vi "S4GUI.vi"(7 "Tab ObsEng":enum32{"Obs", "CCD modes", "Guider", "Eng"}(tab)) -> ()   [LabVIEW 2018] (continued)
                n4865 = Select(t=u8 0, s=w11820, f=u8 6 ("SHUTTER_MODE")) -> (s? t:f=w11821:u8)
              }
            }
          }
          frame Default {
            # "Polar. COM exp mode"
            # "Internal"
            # "Polar. SEM exp mode"
            # "Ext. Start"
            n4866 = Select(t=u8 0, s=w11827, f=u8 6 ("SHUTTER_MODE")) -> (s? t:f=w11824:u8)
          }
        }
        n4867 = call "Write Instrument.lvclass.vi"("error in (no error)"=w11478, "Instrument.lvclass"=w11558, "S4ACS_GUI in"=w11462) -> ("error out"=w11477:errorcluster, "S4ACS_GUI out"=w11466:refnum<class "S4GUI.lvclass">)  [unwired: 7 in]
        n4868 = call-dynamic "Read AcquisitionC.vi"("error in (no error)"=w11477, "S4ACS_GUI in"=w11466) -> ("error out"=w11488:errorcluster, "Acquisition.lvclass"=w11487:refnum<class "Acquisition.lvclass">)  [unwired: 7 in, 1 out]
        n4869 = call-dynamic "Read AcquisitionA.vi"("error in (no error)"=w11477, "S4ACS_GUI in"=w11466) -> ("error out"=w11491:errorcluster, "Acquisition.lvclass"=w11492:refnum<class "Acquisition.lvclass">)  [unwired: 7 in, 1 out]
        n4870 = call "Read AcquisitionB.vi"("error in (no error)"=w11477, "S4ACS_GUI in"=w11466) -> ("error out"=w11489:errorcluster, "Acquisition.lvclass"=w11490:refnum<class "Acquisition.lvclass">)  [unwired: 7 in, 1 out]
        n4871 = call-dynamic "Read AcquisitionD.vi"("error in (no error)"=w11477, "S4ACS_GUI in"=w11466) -> ("error out"=w11485:errorcluster, "Acquisition.lvclass"=w11486:refnum<class "Acquisition.lvclass">)  [unwired: 7 in, 1 out]
        n4872 = call "Read connection.vi"("error in (no error)"=w11488, "Server in"=w11487) -> ("error out"=w11494:errorcluster, "connection"=w11493:bool, "Server out"=w11495:refnum<class "Acquisition.lvclass">)  [unwired: 7 in]
        n4873 = call "Read connection.vi"("error in (no error)"=w11489, "Server in"=w11490) -> ("error out"=w11497:errorcluster, "connection"=w11496:bool, "Server out"=w11498:refnum<class "Acquisition.lvclass">)  [unwired: 7 in]
        n4874 = call "Read connection.vi"("error in (no error)"=w11485, "Server in"=w11486) -> ("error out"=w11474:errorcluster, "connection"=w11475:bool, "Server out"=w11476:refnum<class "Acquisition.lvclass">)  [unwired: 7 in]
        n4875 = call "Read connection.vi"("error in (no error)"=w11491, "Server in"=w11492) -> ("error out"=w11500:errorcluster, "connection"=w11499:bool, "Server out"=w11501:refnum<class "Acquisition.lvclass">)  [unwired: 7 in]
        n4876 = case shown="True" w11493 {
          tunnel: w11495 -> [w11665 w11670]
          tunnel: w11494 -> [w11664 w11669]
          tunnel: [w11665 w11668] -> w11480
          tunnel: [w11664 w11667] -> w11479
          tunnel: w11473 -> [_ w11666]
          frame False {
          }
          frame True {
            # "nome do arquivo .cfg"
            # "seção no arquivo .cfg"
            n4877 = call-dynamic "Read Channel.vi"("error in (no error)"=w11669, "Acquisition in"=w11670) -> ("error out"=w11674:errorcluster, "Channel.lvclass"=w11673:refnum<class "Channel.lvclass">, "Acquisition out"=w11672:refnum<class "Acquisition.lvclass">)  [unwired: 7 in]
            n4878 = call-dynamic "Read Interface.vi"("error in (no error)"=w11674, "Channel in"=w11673) -> ("error out"=w11681:errorcluster, "Interface.lvclass"=w11682:refnum<class "Interface.lvclass">, "Channel out"=w11671:refnum<class "Channel.lvclass">)  [unwired: 7 in]
            n4879 = call-dynamic "Get CCD_Config.vi"("error in (no error)"=w11681, "Interface in"=w11682) -> ("error out"=w11679:errorcluster, "output cluster"=w11678:T31, "Interface out"=w11683:refnum<class "Interface.lvclass">)  [unwired: 7 in]
            n4880 = Bundle By Name(cluster=w11678, "TRIGGER_MODE"=w11666) -> (w11680:T31)
            n4881 = call-dynamic "Set CCD_Config.vi"("error in (no error)"=w11679, "input cluster"=w11680, "Interface in"=w11683) -> ("error out"=w11677:errorcluster, "Interface out"=w11684:refnum<class "Interface.lvclass">)  [unwired: 7 in]
            n4882 = Flatten To String(anything=w11680, error in (no error)=w11677) -> (data string=w11675:string, error out=w11676:errorcluster)  [unwired: 2 in, 1 out]
            n4883 = call "Write flatted cluster.vi"("error in (no error)"=w11676, "flatted cluster"=w11675, "Interface in"=w11684) -> ("error out"=w11686:errorcluster, "Interface out"=w11685:refnum<class "Interface.lvclass">)  [unwired: 7 in]
            n4884 = call-dynamic "Write Interface.vi"("error in (no error)"=w11686, "Interface.lvclass"=w11685, "Channel in"=w11671) -> ("error out"=w11692:errorcluster, "Channel out"=w11693:refnum<class "Channel.lvclass">)  [unwired: 7 in]
            n4885 = call "Write section_name.vi"("error in (no error)"=w11692, "section_name"="CCD_ACS3", "Channel in"=w11693) -> ("error out"=w11690:errorcluster, "Channel out"=w11696:refnum<class "Channel.lvclass">)  [unwired: 7 in]
            n4886 = call-dynamic "save config.vi"("error in (no error)"=w11690, "file config"="lastsaved.cfg", "Channel in"=w11696) -> ("error out"=w11691:errorcluster, "Channel out"=w11697:refnum<class "Channel.lvclass">)  [unwired: 7 in]
            n4887 = call-dynamic "Read State Machine.vi"("error in (no error)"=w11691, "Device in"=w11697) -> ("error out"=w11687:errorcluster, "State Machine.lvclass"=w11699:refnum<class "State Machine.lvclass">, "Device out"=w11698:refnum<class "Channel.lvclass">)  [unwired: 7 in]
            n4888 = call-dynamic "Write State.vi"("error in (no error)"=w11687, "State"=60, "State Machine in"=w11699) -> ("error out"=w11688:errorcluster, "State Machine out"=w11700:refnum<class "State Machine.lvclass">)  [unwired: 7 in]
            n4889 = call-dynamic "Write State Machine.vi"("error in (no error)"=w11688, "State Machine.lvclass"=w11700, "Device in"=w11698) -> ("error out"=w11702:errorcluster, "Device out"=w11701:refnum<class "Channel.lvclass">)  [unwired: 7 in]
            n4890 = call-dynamic "Write Channel.vi"("error in (no error)"=w11702, "Channel.lvclass"=w11701, "Acquisition in"=w11672) -> ("error out"=w11667:errorcluster, "Acquisition out"=w11668:refnum<class "Acquisition.lvclass">)  [unwired: 7 in]
          }
        }
        n4891 = case shown="True" w11475 {
          tunnel: w11476 -> [w11626 w11631]
          tunnel: w11474 -> [w11625 w11630]
          tunnel: w11473 -> [_ w11629]
          tunnel: [w11626 w11628] -> w11472
          tunnel: [w11625 w11627] -> w11471
          frame False {
          }
          frame True {
            # "nome do arquivo .cfg"
            # "seção no arquivo .cfg"
            n4892 = call-dynamic "Read Channel.vi"("error in (no error)"=w11630, "Acquisition in"=w11631) -> ("error out"=w11660:errorcluster, "Channel.lvclass"=w11661:refnum<class "Channel.lvclass">, "Acquisition out"=w11662:refnum<class "Acquisition.lvclass">)  [unwired: 7 in]
            n4893 = call-dynamic "Read Interface.vi"("error in (no error)"=w11660, "Channel in"=w11661) -> ("error out"=w11653:errorcluster, "Interface.lvclass"=w11652:refnum<class "Interface.lvclass">, "Channel out"=w11663:refnum<class "Channel.lvclass">)  [unwired: 7 in]
            n4894 = call-dynamic "Get CCD_Config.vi"("error in (no error)"=w11653, "Interface in"=w11652) -> ("error out"=w11655:errorcluster, "output cluster"=w11656:T31, "Interface out"=w11651:refnum<class "Interface.lvclass">)  [unwired: 7 in]
            n4895 = Bundle By Name(cluster=w11656, "TRIGGER_MODE"=w11629) -> (w11654:T31)
            n4896 = call-dynamic "Set CCD_Config.vi"("error in (no error)"=w11655, "input cluster"=w11654, "Interface in"=w11651) -> ("error out"=w11657:errorcluster, "Interface out"=w11650:refnum<class "Interface.lvclass">)  [unwired: 7 in]
            n4897 = Flatten To String(anything=w11654, error in (no error)=w11657) -> (data string=w11659:string, error out=w11658:errorcluster)  [unwired: 2 in, 1 out]
            n4898 = call "Write flatted cluster.vi"("error in (no error)"=w11658, "flatted cluster"=w11659, "Interface in"=w11650) -> ("error out"=w11648:errorcluster, "Interface out"=w11649:refnum<class "Interface.lvclass">)  [unwired: 7 in]
            n4899 = call-dynamic "Write Interface.vi"("error in (no error)"=w11648, "Interface.lvclass"=w11649, "Channel in"=w11663) -> ("error out"=w11642:errorcluster, "Channel out"=w11641:refnum<class "Channel.lvclass">)  [unwired: 7 in]
            n4900 = call "Write section_name.vi"("error in (no error)"=w11642, "section_name"="CCD_ACS4", "Channel in"=w11641) -> ("error out"=w11644:errorcluster, "Channel out"=w11638:refnum<class "Channel.lvclass">)  [unwired: 7 in]
            n4901 = call-dynamic "save config.vi"("error in (no error)"=w11644, "file config"="lastsaved.cfg", "Channel in"=w11638) -> ("error out"=w11643:errorcluster, "Channel out"=w11637:refnum<class "Channel.lvclass">)  [unwired: 7 in]
            n4902 = call-dynamic "Read State Machine.vi"("error in (no error)"=w11643, "Device in"=w11637) -> ("error out"=w11647:errorcluster, "State Machine.lvclass"=w11635:refnum<class "State Machine.lvclass">, "Device out"=w11636:refnum<class "Channel.lvclass">)  [unwired: 7 in]
            n4903 = call-dynamic "Write State.vi"("error in (no error)"=w11647, "State"=60, "State Machine in"=w11635) -> ("error out"=w11646:errorcluster, "State Machine out"=w11634:refnum<class "State Machine.lvclass">)  [unwired: 7 in]
            n4904 = call-dynamic "Write State Machine.vi"("error in (no error)"=w11646, "State Machine.lvclass"=w11634, "Device in"=w11636) -> ("error out"=w11632:errorcluster, "Device out"=w11633:refnum<class "Channel.lvclass">)  [unwired: 7 in]
            n4905 = call-dynamic "Write Channel.vi"("error in (no error)"=w11632, "Channel.lvclass"=w11633, "Acquisition in"=w11662) -> ("error out"=w11627:errorcluster, "Acquisition out"=w11628:refnum<class "Acquisition.lvclass">)  [unwired: 7 in]
          }
        }
        n4906 = case shown="True" w11496 {
          tunnel: w11498 -> [w11704 w11709]
          tunnel: w11497 -> [w11703 w11708]
          tunnel: [w11704 w11707] -> w11482
          tunnel: [w11703 w11706] -> w11481
          tunnel: w11473 -> [_ w11705]
          frame False {
          }
          frame True {
            # "nome do arquivo .cfg"
            # "seção no arquivo .cfg"
            n4907 = call-dynamic "Read Channel.vi"("error in (no error)"=w11708, "Acquisition in"=w11709) -> ("error out"=w11713:errorcluster, "Channel.lvclass"=w11712:refnum<class "Channel.lvclass">, "Acquisition out"=w11711:refnum<class "Acquisition.lvclass">)  [unwired: 7 in]
            n4908 = call-dynamic "Read Interface.vi"("error in (no error)"=w11713, "Channel in"=w11712) -> ("error out"=w11720:errorcluster, "Interface.lvclass"=w11721:refnum<class "Interface.lvclass">, "Channel out"=w11710:refnum<class "Channel.lvclass">)  [unwired: 7 in]
            n4909 = call-dynamic "Get CCD_Config.vi"("error in (no error)"=w11720, "Interface in"=w11721) -> ("error out"=w11718:errorcluster, "output cluster"=w11717:T31, "Interface out"=w11722:refnum<class "Interface.lvclass">)  [unwired: 7 in]
            n4910 = Bundle By Name(cluster=w11717, "TRIGGER_MODE"=w11705) -> (w11719:T31)
            n4911 = call-dynamic "Set CCD_Config.vi"("error in (no error)"=w11718, "input cluster"=w11719, "Interface in"=w11722) -> ("error out"=w11716:errorcluster, "Interface out"=w11723:refnum<class "Interface.lvclass">)  [unwired: 7 in]
            n4912 = Flatten To String(anything=w11719, error in (no error)=w11716) -> (data string=w11714:string, error out=w11715:errorcluster)  [unwired: 2 in, 1 out]
            n4913 = call "Write flatted cluster.vi"("error in (no error)"=w11715, "flatted cluster"=w11714, "Interface in"=w11723) -> ("error out"=w11725:errorcluster, "Interface out"=w11724:refnum<class "Interface.lvclass">)  [unwired: 7 in]
            n4914 = call-dynamic "Write Interface.vi"("error in (no error)"=w11725, "Interface.lvclass"=w11724, "Channel in"=w11710) -> ("error out"=w11731:errorcluster, "Channel out"=w11732:refnum<class "Channel.lvclass">)  [unwired: 7 in]
            n4915 = call "Write section_name.vi"("error in (no error)"=w11731, "section_name"="CCD_ACS2", "Channel in"=w11732) -> ("error out"=w11729:errorcluster, "Channel out"=w11735:refnum<class "Channel.lvclass">)  [unwired: 7 in]
            n4916 = call-dynamic "save config.vi"("error in (no error)"=w11729, "file config"="lastsaved.cfg", "Channel in"=w11735) -> ("error out"=w11730:errorcluster, "Channel out"=w11736:refnum<class "Channel.lvclass">)  [unwired: 7 in]
            n4917 = call-dynamic "Read State Machine.vi"("error in (no error)"=w11730, "Device in"=w11736) -> ("error out"=w11726:errorcluster, "State Machine.lvclass"=w11738:refnum<class "State Machine.lvclass">, "Device out"=w11737:refnum<class "Channel.lvclass">)  [unwired: 7 in]
            n4918 = call-dynamic "Write State.vi"("error in (no error)"=w11726, "State"=60, "State Machine in"=w11738) -> ("error out"=w11727:errorcluster, "State Machine out"=w11739:refnum<class "State Machine.lvclass">)  [unwired: 7 in]
            n4919 = call-dynamic "Write State Machine.vi"("error in (no error)"=w11727, "State Machine.lvclass"=w11739, "Device in"=w11737) -> ("error out"=w11741:errorcluster, "Device out"=w11740:refnum<class "Channel.lvclass">)  [unwired: 7 in]
            n4920 = call-dynamic "Write Channel.vi"("error in (no error)"=w11741, "Channel.lvclass"=w11740, "Acquisition in"=w11711) -> ("error out"=w11706:errorcluster, "Acquisition out"=w11707:refnum<class "Acquisition.lvclass">)  [unwired: 7 in]
          }
        }
        n4921 = case shown="True" w11499 {
          tunnel: [w11742 w11776] -> w11483
          tunnel: [w11743 w11775] -> w11484
          tunnel: w11501 -> [w11743 w11746]
          tunnel: w11500 -> [w11742 w11745]
          tunnel: w11473 -> [_ w11744]
          frame False {
          }
          frame True {
            # "nome do arquivo .cfg"
            # "seção no arquivo .cfg"
            n4922 = call-dynamic "Read Channel.vi"("error in (no error)"=w11745, "Acquisition in"=w11746) -> ("error out"=w11777:errorcluster, "Channel.lvclass"=w11778:refnum<class "Channel.lvclass">, "Acquisition out"=w11779:refnum<class "Acquisition.lvclass">)  [unwired: 7 in]
            n4923 = call-dynamic "Read Interface.vi"("error in (no error)"=w11777, "Channel in"=w11778) -> ("error out"=w11768:errorcluster, "Interface.lvclass"=w11767:refnum<class "Interface.lvclass">, "Channel out"=w11780:refnum<class "Channel.lvclass">)  [unwired: 7 in]
            n4924 = call-dynamic "Get CCD_Config.vi"("error in (no error)"=w11768, "Interface in"=w11767) -> ("error out"=w11770:errorcluster, "output cluster"=w11771:T31, "Interface out"=w11766:refnum<class "Interface.lvclass">)  [unwired: 7 in]
            n4925 = Bundle By Name(cluster=w11771, "TRIGGER_MODE"=w11744) -> (w11769:T31)
            n4926 = call-dynamic "Set CCD_Config.vi"("error in (no error)"=w11770, "input cluster"=w11769, "Interface in"=w11766) -> ("error out"=w11772:errorcluster, "Interface out"=w11765:refnum<class "Interface.lvclass">)  [unwired: 7 in]
            n4927 = Flatten To String(anything=w11769, error in (no error)=w11772) -> (data string=w11774:string, error out=w11773:errorcluster)  [unwired: 2 in, 1 out]
            n4928 = call "Write flatted cluster.vi"("error in (no error)"=w11773, "flatted cluster"=w11774, "Interface in"=w11765) -> ("error out"=w11763:errorcluster, "Interface out"=w11764:refnum<class "Interface.lvclass">)  [unwired: 7 in]
            n4929 = call-dynamic "Write Interface.vi"("error in (no error)"=w11763, "Interface.lvclass"=w11764, "Channel in"=w11780) -> ("error out"=w11758:errorcluster, "Channel out"=w11757:refnum<class "Channel.lvclass">)  [unwired: 7 in]
            n4930 = call "Write section_name.vi"("error in (no error)"=w11758, "section_name"="CCD_ACS1", "Channel in"=w11757) -> ("error out"=w11759:errorcluster, "Channel out"=w11754:refnum<class "Channel.lvclass">)  [unwired: 7 in]
            n4931 = call-dynamic "save config.vi"("error in (no error)"=w11759, "file config"="lastsaved.cfg", "Channel in"=w11754) -> ("error out"=w11747:errorcluster, "Channel out"=w11748:refnum<class "Channel.lvclass">)  [unwired: 7 in]
            n4932 = call-dynamic "Read State Machine.vi"("error in (no error)"=w11747, "Device in"=w11748) -> ("error out"=w11762:errorcluster, "State Machine.lvclass"=w11752:refnum<class "State Machine.lvclass">, "Device out"=w11753:refnum<class "Channel.lvclass">)  [unwired: 7 in]
            n4933 = call-dynamic "Write State.vi"("error in (no error)"=w11762, "State"=60, "State Machine in"=w11752) -> ("error out"=w11761:errorcluster, "State Machine out"=w11751:refnum<class "State Machine.lvclass">)  [unwired: 7 in]
            n4934 = call-dynamic "Write State Machine.vi"("error in (no error)"=w11761, "State Machine.lvclass"=w11751, "Device in"=w11753) -> ("error out"=w11749:errorcluster, "Device out"=w11750:refnum<class "Channel.lvclass">)  [unwired: 7 in]
            n4935 = call-dynamic "Write Channel.vi"("error in (no error)"=w11749, "Channel.lvclass"=w11750, "Acquisition in"=w11779) -> ("error out"=w11776:errorcluster, "Acquisition out"=w11775:refnum<class "Acquisition.lvclass">)  [unwired: 7 in]
          }
        }
        n4936 = call-dynamic "Write AcquisitionA.vi"("error in (no error)"=w11483, "Acquisition.lvclass"=w11484, "S4ACS_GUI in"=w11466) -> ("error out"=w11470:errorcluster, "S4ACS_GUI out"=w11465:refnum<class "S4GUI.lvclass">)  [unwired: 7 in]
        n4937 = call "Write AcquisitionB.vi"("error in (no error)"=w11481, "Acquisition.lvclass"=w11482, "S4ACS_GUI in"=w11465) -> ("error out"=w11469:errorcluster, "S4ACS_GUI out"=w11464:refnum<class "S4GUI.lvclass">)  [unwired: 7 in]
        n4938 = call-dynamic "Write AcquisitionC.vi"("error in (no error)"=w11479, "Acquisition.lvclass"=w11480, "S4ACS_GUI in"=w11464) -> ("error out"=w11468:errorcluster, "S4ACS_GUI out"=w11463:refnum<class "S4GUI.lvclass">)  [unwired: 7 in]
        n4939 = call-dynamic "Write AcquisitionD.vi"("error in (no error)"=w11471, "Acquisition.lvclass"=w11472, "S4ACS_GUI in"=w11463) -> ("error out"=w11467:errorcluster, "S4ACS_GUI out"=w11447:refnum<class "S4GUI.lvclass">)  [unwired: 7 in]
        n4940 = Merge Errors(w11470, w11469, w11468, w11467) -> (w11446:errorcluster)
        n4941 = call "Read Instrument.lvclass.vi"("error in (no error)"=w11446, "S4ACS_GUI in"=w11447) -> ("error out"=w11452:errorcluster, "Instrument.lvclass"=w11451:refnum<class "Instrument.lvclass">, "S4ACS_GUI out"=w11448:refnum<class "S4GUI.lvclass">)  [unwired: 7 in]
        n4942 = call "Read ASEL.vi"("error in (no error)"=w11452, "Instrument in"=w11451) -> ("error out"=w11459:errorcluster, "Opt_Selector.lvclass"=w11458:refnum<class "Opt_Selector.lvclass">, "Instrument out"=w11457:refnum<class "Instrument.lvclass">)  [unwired: 7 in]
        n4943 = call "Read target name.vi"("error in (no error)"=w11459, "Optics in"=w11458) -> ("error out"=w11455:errorcluster, "target name"=w11435:string, "Optics out"=w11456:refnum<class "Opt_Selector.lvclass">)  [unwired: 7 in]
        n4944 = call "Write ASEL.vi"("error in (no error)"=w11455, "Opt_Selector.lvclass"=w11456, "Instrument in"=w11457) -> ("error out"=w11454:errorcluster, "Instrument out"=w11450:refnum<class "Instrument.lvclass">)  [unwired: 7 in]
        n4945 = Concatenate Strings(w11437, " ASEL=" ("string"), w11435) -> (w11432:string)
        n4946 = case shown="\"ON\"" w11435 {
          tunnel: w11454 -> [w11601 w11612]
          tunnel: [w11601 w11608] -> w11453
          tunnel: w11450 -> [w11600 w11613]
          tunnel: [w11600 w11609] -> w11449
          frame Default {
          }
          frame "ON" {
            n4947 = call "Read WPROT.vi"("error in (no error)"=w11612, "Instrument in"=w11613) -> ("error out"=w11604:errorcluster, "Opt_Selector.lvclass"=w11611:refnum<class "Opt_Selector.lvclass">, "Instrument out"=w11610:refnum<class "Instrument.lvclass">)  [unwired: 7 in]
            n4948 = call-dynamic "Read sequencia.vi"("error in (no error)"=w11604, "Opt_Selector in"=w11611) -> ("error out"=w11603:errorcluster, "sequencia"=w11607:u16, "Opt_Selector out"=w11606:refnum<class "Opt_Selector.lvclass">)  [unwired: 7 in]
            n4949 = case shown="0" w11607 {
              tunnel: w11606 -> [w11615 w11624]
              tunnel: [w11615 w11620] -> w11605
              tunnel: w11603 -> [w11614 w11623]
              tunnel: [w11614 w11618] -> w11602
              frame Default {
              }
              frame 0 {
                n4950 = call-dynamic "Write sequencia.vi"("error in (no error)"=w11623, "sequencia"=u16 1, "Opt_Selector in"=w11624) -> ("error out"=w11619:errorcluster, "Opt_Selector out"=w11621:refnum<class "Opt_Selector.lvclass">)  [unwired: 7 in]
                n4951 = local write "P0"(TRUE ("P0")) -> ()
                n4952 = call-dynamic "Write sequencia_ant.vi"("error in (no error)"=w11619, "sequencia_ant"=u16 1, "Opt_Selector in"=w11621) -> ("error out"=w11618:errorcluster, "Opt_Selector out"=w11620:refnum<class "Opt_Selector.lvclass">)  [unwired: 7 in]
              }
            }
            n4953 = call "Write WPROT.vi"("error in (no error)"=w11602, "Opt_Selector.lvclass"=w11605, "Instrument in"=w11610) -> ("error out"=w11608:errorcluster, "Instrument out"=w11609:refnum<class "Instrument.lvclass">)  [unwired: 7 in]
          }
        }
        n4954 = call "Write Instrument.lvclass.vi"("error in (no error)"=w11453, "Instrument.lvclass"=w11449, "S4ACS_GUI in"=w11448) -> ("error out"=w11433:errorcluster, "S4ACS_GUI out"=w11434:refnum<class "S4GUI.lvclass">)  [unwired: 7 in]
        n4955 = call-dynamic "Write User Event.vi"("error in (no error)"=w11433, "User Event"=w11432, "S4GUI in"=w11434) -> ("error out"=w11430:errorcluster, "S4GUI out"=w11431:refnum<class "S4GUI.lvclass">)  [unwired: 7 in]
      }
      event "Init mode": Value Change {
        n4956 = event-data() -> ()  [unwired: 1 in, 4 out]
        n4957 = call-dynamic "Write User Event.vi"("error in (no error)"=w11833, "User Event"="INIT INSTRUMENT CLICKED", "S4GUI in"=w11834) -> ("error out"=w11831:errorcluster, "S4GUI out"=w11832:refnum<class "S4GUI.lvclass">)  [unwired: 7 in]
        n4958 = call-dynamic "Read Obs_state.vi"("error in (no error)"=w11831, "S4ACS_GUI in"=w11832) -> ("error out"=w11835:errorcluster, "Obs_state"=w11837:u32, "S4ACS_GUI out"=w11838:refnum<class "S4GUI.lvclass">)  [unwired: 7 in]
        n4959 = In Range and Coerce(upper limit=u32 226, x=w11837, lower limit=u32 220 ("upper limit")) -> (In Range?=w11836:bool)  [unwired: 1 out]
        n4960 = case shown="False" w11836 {
          tunnel: [w11846 w11854] -> w11842
          tunnel: [w11845 w11852] -> w11841
          tunnel: w11835 -> [w11844 w11853]
          tunnel: w11838 -> [w11843 w11855]
          frame False {
            n4961 = call-dynamic "Write sync.vi"("error in (no error)"=w11844, "sync"=TRUE, "S4ACS_GUI in"=w11843) -> ("error out"=w11848:errorcluster, "S4ACS_GUI out"=w11847:refnum<class "S4GUI.lvclass">)  [unwired: 7 in]
            n4962 = call-dynamic "Write Obs_state.vi"("error in (no error)"=w11848, "Obs_state"=u32 220, "S4ACS_GUI in"=w11847) -> ("error out"=w11845:errorcluster, "S4ACS_GUI out"=w11846:refnum<class "S4GUI.lvclass">)  [unwired: 7 in]
          }
          frame True {
            n4963 = call-dynamic "Write Obs_state.vi"("error in (no error)"=w11853, "Obs_state"=u32 0, "S4ACS_GUI in"=w11855) -> ("error out"=w11852:errorcluster, "S4ACS_GUI out"=w11854:refnum<class "S4GUI.lvclass">)  [unwired: 7 in]
          }
        }
      }
      event "exit": Value Change {
        n4964 = event-data() -> ()  [unwired: 1 in, 4 out]
        n4965 = call-dynamic "Read Obs_state.vi"("error in (no error)"=w11859, "S4ACS_GUI in"=w11860) -> ("error out"=w11857:errorcluster, "Obs_state"=w11861:u32, "S4ACS_GUI out"=w11858:refnum<class "S4GUI.lvclass">)  [unwired: 7 in]
        n4966 = In Range and Coerce(upper limit=u32 239, x=w11861, lower limit=u32 230 ("upper limit")) -> (In Range?=w11856:bool)  [unwired: 1 out]
        n4967 = case shown="False" w11856 {
          tunnel: [w11874 w12006] -> w11865
          tunnel: [w11873 w12005] -> w11864
          tunnel: w11858 -> [w11867 w12006]
          tunnel: w11857 -> [w11866 w12005]
          frame False {
            n4968 = call "Read Instrument.lvclass.vi"("error in (no error)"=w11866, "S4ACS_GUI in"=w11867) -> ("error out"=w11868:errorcluster, "Instrument.lvclass"=w11870:refnum<class "Instrument.lvclass">, "S4ACS_GUI out"=w11872:refnum<class "S4GUI.lvclass">)  [unwired: 7 in]
            n4969 = call-dynamic "Read operational.vi"("error in (no error)"=w11868, "Server in"=w11870) -> ("error out"=w11871:errorcluster, "operational"=w11869:bool)  [unwired: 7 in, 1 out]
            n4970 = case shown="True" w11869 {
              tunnel: [w11884 w11952] -> w11874
              tunnel: [w11883 w11951] -> w11873
              tunnel: w11872 -> [w11881 w11950]
              tunnel: w11871 -> [w11882 w11949]
              frame False {
                # "Park condition:\nidle: T\nAND\nall discon: F"
                # "S4ICS not operational: only ACS parking can \nbe allowed, depending on its status..."
                n4971 = call-dynamic "VerifyAcqStatus.vi"("error in (no error)"=w11882, "S4GUI in"=w11881) -> ("error out"=w11876:errorcluster, "idle"=w11880:bool, "S4GUI out"=w11878:refnum<class "S4GUI.lvclass">)  [unwired: 6 in, 1 out]
                n4972 = case shown="True" w11880 {
                  selector: w11880 -> [w11885 _]
                  tunnel: [w11885 w11888] -> w11879
                  tunnel: w11878 -> [w11887 w11892]
                  tunnel: [w11887 w11891] -> w11877
                  tunnel: w11876 -> [w11886 w11890]
                  tunnel: [w11886 w11889] -> w11875
                  frame False {
                  }
                  frame True {
                    n4973 = call-dynamic "VerifAllChanDiscon.vi"("error in (no error)"=w11890, "S4GUI in"=w11892) -> ("error out"=w11889:errorcluster, "All disconnected"=w11893:bool, "S4GUI out"=w11891:refnum<class "S4GUI.lvclass">)  [unwired: 7 in]
                    n4974 = Not(x=w11893) -> (.not. x?=w11888:bool)
                  }
                }
                n4975 = case shown="False" w11879 {
                  tunnel: w11875 -> [w11902 w11921]
                  tunnel: w11877 -> [w11903 w11920]
                  tunnel: [w11896 w11919] -> w11884
                  tunnel: [w11895 w11918] -> w11883
                  frame False {
                    # "Acquisition in progress OR no channel operational..."
                    n4976 = Two Button Dialog(message="Parking not possible.\nAre you sure to quit?", 2:"Yes" ("T button name (\"OK\")")) -> (T button?=w11899:bool)  [unwired: 1 in]
                    n4977 = case shown="True" w11899 {
                      tunnel: [w11906 w11910] -> w11898
                      tunnel: w11903 -> [w11906 w11911]
                      tunnel: w11902 -> [w11905 w11909]
                      tunnel: [w11905 w11908] -> w11897
                      tunnel: ["EXIT CLICKED WITH NO PARKING POSSIBLE. EXIT CANCELLED. " ("T button name (\"OK\")") "EXIT CLICKED WITH NO PARKING POSSIBLE." ("T button name (\"OK\")")] -> w11894
                      frame False {
                        # "NO (cancel)"
                      }
                      frame True {
                        # "YES"
                        n4978 = call-dynamic "Write exit.vi"("error in (no error)"=w11909, "exit"=TRUE, "S4GUI in"=w11911) -> ("error out"=w11908:errorcluster, "S4GUI out"=w11910:refnum<class "S4GUI.lvclass">)  [unwired: 7 in]
                      }
                    }
                    n4979 = call-dynamic "Write User Event.vi"("error in (no error)"=w11897, "User Event"=w11894, "S4GUI in"=w11898) -> ("error out"=w11895:errorcluster, "S4GUI out"=w11896:refnum<class "S4GUI.lvclass">)  [unwired: 7 in]
                  }
                  frame True {
                    # "No acquisition in progress."
                    n4980 = call <vilib>:"Three Button Dialog.vi"("Right Button Text (\"Cancel\")"="Cancel" ("Right Button Text (\"Cancel\")"), "Center Button Text (\"No\")"="NO" ("F button name (\"Cancel\")"), "Left Button Text (\"Yes\")"="YES" ("T button name (\"OK\")"), "message"="Instrument parking not possible.\nPark acquisition system before exiting?") -> ("Which Button?"=w11916:T34)  [unwired: 7 in]
                    n4981 = case shown="\"Right Button\", Default" w11916 {
                      tunnel: w11921 -> [w11928 w11932 w11941]
                      tunnel: w11920 -> [w11927 w11933 w11940]
                      tunnel: [w11924 w11931 w11937] -> w11919
                      tunnel: [w11922 w11930 w11935] -> w11918
                      frame "Center Button" {
                        # "NO"
                        n4982 = call-dynamic "Write exit.vi"("error in (no error)"=w11928, "exit"=TRUE, "S4GUI in"=w11927) -> ("error out"=w11923:errorcluster, "S4GUI out"=w11925:refnum<class "S4GUI.lvclass">)  [unwired: 7 in]
                        n4983 = call-dynamic "Write User Event.vi"("error in (no error)"=w11923, "User Event"="EXIT APP CLICKED WITH NO PARKING.", "S4GUI in"=w11925) -> ("error out"=w11922:errorcluster, "S4GUI out"=w11924:refnum<class "S4GUI.lvclass">)  [unwired: 7 in]
                      }
                      frame "Right Button", Default {
                        # "CANCEL"
                        n4984 = call-dynamic "Write User Event.vi"("error in (no error)"=w11932, "User Event"="EXIT APP CLICKED, BUT CANCELLED BY USER.", "S4GUI in"=w11933) -> ("error out"=w11930:errorcluster, "S4GUI out"=w11931:refnum<class "S4GUI.lvclass">)  [unwired: 7 in]
                      }
                      frame "Left Button" {
                        # "YES"
                        n4985 = call-dynamic "Write sync.vi"("error in (no error)"=w11941, "sync"=TRUE, "S4ACS_GUI in"=w11940) -> ("error out"=w11943:errorcluster, "S4ACS_GUI out"=w11942:refnum<class "S4GUI.lvclass">)  [unwired: 7 in]
                        n4986 = call-dynamic "Write Obs_state.vi"("error in (no error)"=w11943, "Obs_state"=u32 232, "S4ACS_GUI in"=w11942) -> ("error out"=w11936:errorcluster, "S4ACS_GUI out"=w11938:refnum<class "S4GUI.lvclass">)  [unwired: 7 in]
                        n4987 = call-dynamic "Write User Event.vi"("error in (no error)"=w11936, "User Event"="EXIT APP CLICKED AND ONLY ACS PARKING PROCEDURE DONE.", "S4GUI in"=w11938) -> ("error out"=w11935:errorcluster, "S4GUI out"=w11937:refnum<class "S4GUI.lvclass">)  [unwired: 7 in]
                      }
                    }
                  }
                }
              }
              frame True {
                # "Park condition:\nidle: T"
                # "S4ICS operational: Instrument parking allowed \nand verifying ACS channels status..."
                n4988 = call-dynamic "VerifyAcqStatus.vi"("error in (no error)"=w11949, "S4GUI in"=w11950) -> ("error out"=w11946:errorcluster, "idle"=w11947:bool, "S4GUI out"=w11948:refnum<class "S4GUI.lvclass">)  [unwired: 6 in, 1 out]
                n4989 = case shown="False" w11947 {
                  tunnel: [w11956 w11980] -> w11952
                  tunnel: [w11955 w11979] -> w11951
                  tunnel: w11948 -> [w11954 w11973]
                  tunnel: w11946 -> [w11953 w11972]
                  frame False {
                    # "Acquisition in progress..."
                    n4990 = Two Button Dialog(message="Parking not possible.\nAre you sure to quit?", 2:"Yes" ("T button name (\"OK\")")) -> (T button?=w11960:bool)  [unwired: 1 in]
                    n4991 = case shown="True" w11960 {
                      tunnel: [w11965 w11969] -> w11959
                      tunnel: w11954 -> [w11965 w11970]
                      tunnel: w11953 -> [w11964 w11968]
                      tunnel: [w11964 w11967] -> w11958
                      tunnel: ["EXIT CLICKED WITH NO PARKING POSSIBLE. EXIT CANCELLED. " ("T button name (\"OK\")") "EXIT CLICKED WITH NO PARKING POSSIBLE." ("T button name (\"OK\")")] -> w11957
                      frame False {
                        # "NO (cancel)"
                      }
                      frame True {
                        # "YES"
                        n4992 = call-dynamic "Write exit.vi"("error in (no error)"=w11968, "exit"=TRUE, "S4GUI in"=w11970) -> ("error out"=w11967:errorcluster, "S4GUI out"=w11969:refnum<class "S4GUI.lvclass">)  [unwired: 7 in]
                      }
                    }
                    n4993 = call-dynamic "Write User Event.vi"("error in (no error)"=w11958, "User Event"=w11957, "S4GUI in"=w11959) -> ("error out"=w11955:errorcluster, "S4GUI out"=w11956:refnum<class "S4GUI.lvclass">)  [unwired: 7 in]
                  }
                  frame True {
                    # "Acquisition system in IDLE state."
                    n4994 = call <vilib>:"Three Button Dialog.vi"("Right Button Text (\"Cancel\")"="Cancel" ("Right Button Text (\"Cancel\")"), "Center Button Text (\"No\")"="NO" ("F button name (\"Cancel\")"), "Left Button Text (\"Yes\")"="YES" ("T button name (\"OK\")"), "message"="Park before exiting?") -> ("Which Button?"=w11975:T34)  [unwired: 7 in]
                    n4995 = case shown="\"Left Button\"" w11975 {
                      tunnel: w11972 -> [w11987 w11991 w12001]
                      tunnel: w11973 -> [w11986 w11992 w12000]
                      tunnel: [w11983 w11990 w11997] -> w11980
                      tunnel: [w11981 w11989 w11995] -> w11979
                      frame "Center Button" {
                        # "NO"
                        n4996 = call-dynamic "Write exit.vi"("error in (no error)"=w11987, "exit"=TRUE, "S4GUI in"=w11986) -> ("error out"=w11982:errorcluster, "S4GUI out"=w11984:refnum<class "S4GUI.lvclass">)  [unwired: 7 in]
                        n4997 = call-dynamic "Write User Event.vi"("error in (no error)"=w11982, "User Event"="EXIT APP CLICKED WITH NO PARKING.", "S4GUI in"=w11984) -> ("error out"=w11981:errorcluster, "S4GUI out"=w11983:refnum<class "S4GUI.lvclass">)  [unwired: 7 in]
                      }
                      frame "Right Button", Default {
                        # "CANCEL"
                        n4998 = call-dynamic "Write User Event.vi"("error in (no error)"=w11991, "User Event"="EXIT APP CLICKED, BUT CANCELLED BY USER.", "S4GUI in"=w11992) -> ("error out"=w11989:errorcluster, "S4GUI out"=w11990:refnum<class "S4GUI.lvclass">)  [unwired: 7 in]
                      }
                      frame "Left Button" {
                        # "YES"
                        n4999 = call-dynamic "Write sync.vi"("error in (no error)"=w12001, "sync"=TRUE, "S4ACS_GUI in"=w12000) -> ("error out"=w12003:errorcluster, "S4ACS_GUI out"=w12002:refnum<class "S4GUI.lvclass">)  [unwired: 7 in]
                        n5000 = call-dynamic "Write Obs_state.vi"("error in (no error)"=w12003, "Obs_state"=u32 230, "S4ACS_GUI in"=w12002) -> ("error out"=w11996:errorcluster, "S4ACS_GUI out"=w11998:refnum<class "S4GUI.lvclass">)  [unwired: 7 in]
                        n5001 = call-dynamic "Write User Event.vi"("error in (no error)"=w11996, "User Event"="EXIT APP CLICKED AND PARKING PROCEDURE DONE.", "S4GUI in"=w11998) -> ("error out"=w11995:errorcluster, "S4GUI out"=w11997:refnum<class "S4GUI.lvclass">)  [unwired: 7 in]
                      }
                    }
                  }
                }
              }
            }
          }
          frame True {
            # "Parking already in progress..."
          }
        }
      }
      event "WPSEL_stop": Value Change {
        n5002 = event-data() -> ()  [unwired: 1 in, 4 out]
        n5003 = call "Read Instrument.lvclass.vi"("error in (no error)"=w12025, "S4ACS_GUI in"=w12026) -> ("error out"=w12023:errorcluster, "Instrument.lvclass"=w12024:refnum<class "Instrument.lvclass">, "S4ACS_GUI out"=w12010:refnum<class "S4GUI.lvclass">)  [unwired: 7 in]
        n5004 = call "Read WPSEL.vi"("error in (no error)"=w12023, "Instrument in"=w12024) -> ("error out"=w12019:errorcluster, "Opt_Selector.lvclass"=w12022:refnum<class "Opt_Selector.lvclass">, "Instrument out"=w12013:refnum<class "Instrument.lvclass">)  [unwired: 7 in]
        n5005 = call-dynamic "Read State Machine.vi"("error in (no error)"=w12019, "Device in"=w12022) -> ("error out"=w12018:errorcluster, "State Machine.lvclass"=w12021:refnum<class "State Machine.lvclass">, "Device out"=w12015:refnum<class "Opt_Selector.lvclass">)  [unwired: 7 in]
        n5006 = call "Next State.vi"("error in (no error)"=w12018, "New_State"=10, "State Machine in"=w12021) -> ("error out"=w12017:errorcluster, "State Machine out"=w12016:refnum<class "State Machine.lvclass">)  [unwired: 7 in]
        n5007 = call-dynamic "Write State Machine.vi"("error in (no error)"=w12017, "State Machine.lvclass"=w12016, "Device in"=w12015) -> ("error out"=w12012:errorcluster, "Device out"=w12014:refnum<class "Opt_Selector.lvclass">)  [unwired: 7 in]
        n5008 = call "Write WPSEL.vi"("error in (no error)"=w12012, "Opt_Selector.lvclass"=w12014, "Instrument in"=w12013) -> ("error out"=w12009:errorcluster, "Instrument out"=w12011:refnum<class "Instrument.lvclass">)  [unwired: 7 in]
        n5009 = call "Write Instrument.lvclass.vi"("error in (no error)"=w12009, "Instrument.lvclass"=w12011, "S4ACS_GUI in"=w12010) -> ("error out"=w12008:errorcluster, "S4ACS_GUI out"=w12007:refnum<class "S4GUI.lvclass">)  [unwired: 7 in]
      }
      event "WPSEL_init": Value Change {
        n5010 = event-data() -> ()  [unwired: 1 in, 4 out]
        n5011 = call "Read Instrument.lvclass.vi"("error in (no error)"=w12045, "S4ACS_GUI in"=w12046) -> ("error out"=w12043:errorcluster, "Instrument.lvclass"=w12044:refnum<class "Instrument.lvclass">, "S4ACS_GUI out"=w12030:refnum<class "S4GUI.lvclass">)  [unwired: 7 in]
        n5012 = call "Read WPSEL.vi"("error in (no error)"=w12043, "Instrument in"=w12044) -> ("error out"=w12039:errorcluster, "Opt_Selector.lvclass"=w12042:refnum<class "Opt_Selector.lvclass">, "Instrument out"=w12033:refnum<class "Instrument.lvclass">)  [unwired: 7 in]
        n5013 = call-dynamic "Read State Machine.vi"("error in (no error)"=w12039, "Device in"=w12042) -> ("error out"=w12038:errorcluster, "State Machine.lvclass"=w12041:refnum<class "State Machine.lvclass">, "Device out"=w12035:refnum<class "Opt_Selector.lvclass">)  [unwired: 7 in]
        n5014 = call "Next State.vi"("error in (no error)"=w12038, "New_State"=30, "State Machine in"=w12041) -> ("error out"=w12037:errorcluster, "State Machine out"=w12036:refnum<class "State Machine.lvclass">)  [unwired: 7 in]
        n5015 = call-dynamic "Write State Machine.vi"("error in (no error)"=w12037, "State Machine.lvclass"=w12036, "Device in"=w12035) -> ("error out"=w12032:errorcluster, "Device out"=w12034:refnum<class "Opt_Selector.lvclass">)  [unwired: 7 in]
        n5016 = call "Write WPSEL.vi"("error in (no error)"=w12032, "Opt_Selector.lvclass"=w12034, "Instrument in"=w12033) -> ("error out"=w12029:errorcluster, "Instrument out"=w12031:refnum<class "Instrument.lvclass">)  [unwired: 7 in]
        n5017 = call "Write Instrument.lvclass.vi"("error in (no error)"=w12029, "Instrument.lvclass"=w12031, "S4ACS_GUI in"=w12030) -> ("error out"=w12028:errorcluster, "S4ACS_GUI out"=w12027:refnum<class "S4GUI.lvclass">)  [unwired: 7 in]
      }
      event "GMIR_target": Value Change {
        n5018 = event-data() -> ("NewVal"=w12056:dbl)  [unwired: 1 in, 3 out]
        n5019 = call "Read Instrument.lvclass.vi"("error in (no error)"=w12060, "S4ACS_GUI in"=w12061) -> ("error out"=w12058:errorcluster, "Instrument.lvclass"=w12059:refnum<class "Instrument.lvclass">, "S4ACS_GUI out"=w12050:refnum<class "S4GUI.lvclass">)  [unwired: 7 in]
        n5020 = call "Read GMIR.vi"("error in (no error)"=w12058, "Instrument in"=w12059) -> ("error out"=w12055:errorcluster, "Opt_Continuous.lvclass"=w12057:refnum<class "Opt_Continuous.lvclass">, "Instrument out"=w12053:refnum<class "Instrument.lvclass">)  [unwired: 7 in]
        n5021 = call "Write target.vi"("error in (no error)"=w12055, "target"=w12056, "Optics in"=w12057) -> ("error out"=w12052:errorcluster, "Optics out"=w12054:refnum<class "Opt_Continuous.lvclass">)  [unwired: 7 in]
        n5022 = call "Write GMIR.vi"("error in (no error)"=w12052, "Opt_Continuous.lvclass"=w12054, "Instrument in"=w12053) -> ("error out"=w12049:errorcluster, "Instrument out"=w12051:refnum<class "Instrument.lvclass">)  [unwired: 7 in]
        n5023 = call "Write Instrument.lvclass.vi"("error in (no error)"=w12049, "Instrument.lvclass"=w12051, "S4ACS_GUI in"=w12050) -> ("error out"=w12048:errorcluster, "S4ACS_GUI out"=w12047:refnum<class "S4GUI.lvclass">)  [unwired: 7 in]
      }
      event "GMIR_target 2": Value Change {
        n5024 = event-data() -> ("NewVal"=w12063:dbl)  [unwired: 1 in, 3 out]
        n5025 = call-dynamic "Read GSserver.lvclass.vi"("error in (no error)"=w12076, "S4GUI in"=w12077) -> ("error out"=w12074:errorcluster, "GSserver.lvclass"=w12075:refnum<class "GSserver.lvclass">, "S4GUI out"=w12071:refnum<class "S4GUI.lvclass">)  [unwired: 7 in]
        n5026 = call-dynamic "Read Mirror.vi"("error in (no error)"=w12074, "GSserver in"=w12075) -> ("error out"=w12065:errorcluster, "GSdevice.lvclass"=w12067:refnum<class "GSdevice.lvclass">, "GSserver out"=w12073:refnum<class "GSserver.lvclass">)  [unwired: 7 in]
        n5027 = Number To Fractional String(number=w12063) -> (F-format string=w12062:string)  [unwired: 3 in]
        n5028 = call-dynamic "Write target.vi"("error in (no error)"=w12065, "target"=w12062, "GSdevice in"=w12067) -> ("error out"=w12064:errorcluster, "GSdevice out"=w12066:refnum<class "GSdevice.lvclass">)  [unwired: 7 in]
        n5029 = call-dynamic "Write Mirror.vi"("error in (no error)"=w12064, "GSdevice.lvclass"=w12066, "GSserver in"=w12073) -> ("error out"=w12070:errorcluster, "GSserver out"=w12072:refnum<class "GSserver.lvclass">)  [unwired: 7 in]
        n5030 = call-dynamic "Write GSserver.lvclass.vi"("error in (no error)"=w12070, "GSserver.lvclass"=w12072, "S4GUI in"=w12071) -> ("error out"=w12069:errorcluster, "S4GUI out"=w12068:refnum<class "S4GUI.lvclass">)  [unwired: 7 in]
      }
      event "GMIR_set": Value Change {
        n5031 = event-data() -> ()  [unwired: 1 in, 4 out]
        n5032 = call "Read Instrument.lvclass.vi"("error in (no error)"=w12096, "S4ACS_GUI in"=w12097) -> ("error out"=w12094:errorcluster, "Instrument.lvclass"=w12095:refnum<class "Instrument.lvclass">, "S4ACS_GUI out"=w12083:refnum<class "S4GUI.lvclass">)  [unwired: 7 in]
        n5033 = call "Read GMIR.vi"("error in (no error)"=w12094, "Instrument in"=w12095) -> ("error out"=w12091:errorcluster, "Opt_Continuous.lvclass"=w12093:refnum<class "Opt_Continuous.lvclass">, "Instrument out"=w12085:refnum<class "Instrument.lvclass">)  [unwired: 7 in]
        n5034 = call-dynamic "Read State Machine.vi"("error in (no error)"=w12091, "Device in"=w12093) -> ("error out"=w12090:errorcluster, "State Machine.lvclass"=w12081:refnum<class "State Machine.lvclass">, "Device out"=w12087:refnum<class "Opt_Continuous.lvclass">)  [unwired: 7 in]
        n5035 = call "Next State.vi"("error in (no error)"=w12090, "New_State"=1, "State Machine in"=w12081) -> ("error out"=w12089:errorcluster, "State Machine out"=w12088:refnum<class "State Machine.lvclass">)  [unwired: 7 in]
        n5036 = call-dynamic "Write State Machine.vi"("error in (no error)"=w12089, "State Machine.lvclass"=w12088, "Device in"=w12087) -> ("error out"=w12084:errorcluster, "Device out"=w12086:refnum<class "Opt_Continuous.lvclass">)  [unwired: 7 in]
        n5037 = call "Write GMIR.vi"("error in (no error)"=w12084, "Opt_Continuous.lvclass"=w12086, "Instrument in"=w12085) -> ("error out"=w12078:errorcluster, "Instrument out"=w12079:refnum<class "Instrument.lvclass">)  [unwired: 7 in]
        n5038 = call "Write Instrument.lvclass.vi"("error in (no error)"=w12078, "Instrument.lvclass"=w12079, "S4ACS_GUI in"=w12083) -> ("error out"=w12082:errorcluster, "S4ACS_GUI out"=w12080:refnum<class "S4GUI.lvclass">)  [unwired: 7 in]
      }
      event "GMIR_set 2": Value Change {
        n5039 = event-data() -> ()  [unwired: 1 in, 4 out]
        n5040 = call-dynamic "Read GSserver.lvclass.vi"("error in (no error)"=w12116, "S4GUI in"=w12117) -> ("error out"=w12114:errorcluster, "GSserver.lvclass"=w12115:refnum<class "GSserver.lvclass">, "S4GUI out"=w12103:refnum<class "S4GUI.lvclass">)  [unwired: 7 in]
        n5041 = call-dynamic "Read Mirror.vi"("error in (no error)"=w12114, "GSserver in"=w12115) -> ("error out"=w12111:errorcluster, "GSdevice.lvclass"=w12113:refnum<class "GSdevice.lvclass">, "GSserver out"=w12105:refnum<class "GSserver.lvclass">)  [unwired: 7 in]
        n5042 = call-dynamic "Read State Machine.vi"("error in (no error)"=w12111, "Device in"=w12113) -> ("error out"=w12110:errorcluster, "State Machine.lvclass"=w12101:refnum<class "State Machine.lvclass">, "Device out"=w12107:refnum<class "GSdevice.lvclass">)  [unwired: 7 in]
        n5043 = call "Next State.vi"("error in (no error)"=w12110, "New_State"=10, "State Machine in"=w12101) -> ("error out"=w12109:errorcluster, "State Machine out"=w12108:refnum<class "State Machine.lvclass">)  [unwired: 7 in]
        n5044 = call-dynamic "Write State Machine.vi"("error in (no error)"=w12109, "State Machine.lvclass"=w12108, "Device in"=w12107) -> ("error out"=w12104:errorcluster, "Device out"=w12106:refnum<class "GSdevice.lvclass">)  [unwired: 7 in]
        n5045 = call-dynamic "Write Mirror.vi"("error in (no error)"=w12104, "GSdevice.lvclass"=w12106, "GSserver in"=w12105) -> ("error out"=w12098:errorcluster, "GSserver out"=w12099:refnum<class "GSserver.lvclass">)  [unwired: 7 in]
        n5046 = call-dynamic "Write GSserver.lvclass.vi"("error in (no error)"=w12098, "GSserver.lvclass"=w12099, "S4GUI in"=w12103) -> ("error out"=w12102:errorcluster, "S4GUI out"=w12100:refnum<class "S4GUI.lvclass">)  [unwired: 7 in]
      }
      event "GMIR_stop", "GMIR_stop 2": Value Change {
        n5047 = event-data() -> ()  [unwired: 1 in, 4 out]
        n5048 = call "Read Instrument.lvclass.vi"("error in (no error)"=w12136, "S4ACS_GUI in"=w12137) -> ("error out"=w12134:errorcluster, "Instrument.lvclass"=w12135:refnum<class "Instrument.lvclass">, "S4ACS_GUI out"=w12121:refnum<class "S4GUI.lvclass">)  [unwired: 7 in]
        n5049 = call "Read GMIR.vi"("error in (no error)"=w12134, "Instrument in"=w12135) -> ("error out"=w12130:errorcluster, "Opt_Continuous.lvclass"=w12133:refnum<class "Opt_Continuous.lvclass">, "Instrument out"=w12124:refnum<class "Instrument.lvclass">)  [unwired: 7 in]
        n5050 = call-dynamic "Read State Machine.vi"("error in (no error)"=w12130, "Device in"=w12133) -> ("error out"=w12129:errorcluster, "State Machine.lvclass"=w12132:refnum<class "State Machine.lvclass">, "Device out"=w12126:refnum<class "Opt_Continuous.lvclass">)  [unwired: 7 in]
        n5051 = call "Next State.vi"("error in (no error)"=w12129, "New_State"=10, "State Machine in"=w12132) -> ("error out"=w12128:errorcluster, "State Machine out"=w12127:refnum<class "State Machine.lvclass">)  [unwired: 7 in]
        n5052 = call-dynamic "Write State Machine.vi"("error in (no error)"=w12128, "State Machine.lvclass"=w12127, "Device in"=w12126) -> ("error out"=w12123:errorcluster, "Device out"=w12125:refnum<class "Opt_Continuous.lvclass">)  [unwired: 7 in]
        n5053 = call "Write GMIR.vi"("error in (no error)"=w12123, "Opt_Continuous.lvclass"=w12125, "Instrument in"=w12124) -> ("error out"=w12120:errorcluster, "Instrument out"=w12122:refnum<class "Instrument.lvclass">)  [unwired: 7 in]
        n5054 = call "Write Instrument.lvclass.vi"("error in (no error)"=w12120, "Instrument.lvclass"=w12122, "S4ACS_GUI in"=w12121) -> ("error out"=w12119:errorcluster, "S4ACS_GUI out"=w12118:refnum<class "S4GUI.lvclass">)  [unwired: 7 in]
      }
      event "GMIR_init": Value Change {
        n5055 = event-data() -> ()  [unwired: 1 in, 4 out]
        n5056 = call "Read Instrument.lvclass.vi"("error in (no error)"=w12156, "S4ACS_GUI in"=w12157) -> ("error out"=w12154:errorcluster, "Instrument.lvclass"=w12155:refnum<class "Instrument.lvclass">, "S4ACS_GUI out"=w12141:refnum<class "S4GUI.lvclass">)  [unwired: 7 in]
        n5057 = call "Read GMIR.vi"("error in (no error)"=w12154, "Instrument in"=w12155) -> ("error out"=w12150:errorcluster, "Opt_Continuous.lvclass"=w12153:refnum<class "Opt_Continuous.lvclass">, "Instrument out"=w12144:refnum<class "Instrument.lvclass">)  [unwired: 7 in]
        n5058 = call-dynamic "Read State Machine.vi"("error in (no error)"=w12150, "Device in"=w12153) -> ("error out"=w12149:errorcluster, "State Machine.lvclass"=w12152:refnum<class "State Machine.lvclass">, "Device out"=w12146:refnum<class "Opt_Continuous.lvclass">)  [unwired: 7 in]
        n5059 = call "Next State.vi"("error in (no error)"=w12149, "New_State"=30, "State Machine in"=w12152) -> ("error out"=w12148:errorcluster, "State Machine out"=w12147:refnum<class "State Machine.lvclass">)  [unwired: 7 in]
        n5060 = call-dynamic "Write State Machine.vi"("error in (no error)"=w12148, "State Machine.lvclass"=w12147, "Device in"=w12146) -> ("error out"=w12143:errorcluster, "Device out"=w12145:refnum<class "Opt_Continuous.lvclass">)  [unwired: 7 in]
        n5061 = call "Write GMIR.vi"("error in (no error)"=w12143, "Opt_Continuous.lvclass"=w12145, "Instrument in"=w12144) -> ("error out"=w12140:errorcluster, "Instrument out"=w12142:refnum<class "Instrument.lvclass">)  [unwired: 7 in]
        n5062 = call "Write Instrument.lvclass.vi"("error in (no error)"=w12140, "Instrument.lvclass"=w12142, "S4ACS_GUI in"=w12141) -> ("error out"=w12139:errorcluster, "S4ACS_GUI out"=w12138:refnum<class "S4GUI.lvclass">)  [unwired: 7 in]
      }
      event "GFOC_target": Value Change {
        n5063 = event-data() -> ("NewVal"=w12167:dbl)  [unwired: 1 in, 3 out]
        n5064 = call "Read Instrument.lvclass.vi"("error in (no error)"=w12171, "S4ACS_GUI in"=w12172) -> ("error out"=w12169:errorcluster, "Instrument.lvclass"=w12170:refnum<class "Instrument.lvclass">, "S4ACS_GUI out"=w12161:refnum<class "S4GUI.lvclass">)  [unwired: 7 in]
        n5065 = call "Read GFOC.vi"("error in (no error)"=w12169, "Instrument in"=w12170) -> ("error out"=w12166:errorcluster, "Opt_Continuous.lvclass"=w12168:refnum<class "Opt_Continuous.lvclass">, "Instrument out"=w12164:refnum<class "Instrument.lvclass">)  [unwired: 7 in]
        n5066 = call "Write target.vi"("error in (no error)"=w12166, "target"=w12167, "Optics in"=w12168) -> ("error out"=w12163:errorcluster, "Optics out"=w12165:refnum<class "Opt_Continuous.lvclass">)  [unwired: 7 in]
        n5067 = call "Write GFOC.vi"("error in (no error)"=w12163, "Opt_Continuous.lvclass"=w12165, "Instrument in"=w12164) -> ("error out"=w12160:errorcluster, "Instrument out"=w12162:refnum<class "Instrument.lvclass">)  [unwired: 7 in]
        n5068 = call "Write Instrument.lvclass.vi"("error in (no error)"=w12160, "Instrument.lvclass"=w12162, "S4ACS_GUI in"=w12161) -> ("error out"=w12159:errorcluster, "S4ACS_GUI out"=w12158:refnum<class "S4GUI.lvclass">)  [unwired: 7 in]
      }
      event "GFOC_target 2": Value Change {
        n5069 = event-data() -> ("NewVal"=w12174:dbl)  [unwired: 1 in, 3 out]
        n5070 = call-dynamic "Read GSserver.lvclass.vi"("error in (no error)"=w12187, "S4GUI in"=w12188) -> ("error out"=w12185:errorcluster, "GSserver.lvclass"=w12186:refnum<class "GSserver.lvclass">, "S4GUI out"=w12178:refnum<class "S4GUI.lvclass">)  [unwired: 7 in]
        n5071 = call-dynamic "Read Focus.vi"("error in (no error)"=w12185, "GSserver in"=w12186) -> ("error out"=w12183:errorcluster, "GSdevice.lvclass"=w12184:refnum<class "GSdevice.lvclass">, "GSserver out"=w12181:refnum<class "GSserver.lvclass">)  [unwired: 7 in]
        n5072 = Number To Fractional String(number=w12174) -> (F-format string=w12173:string)  [unwired: 3 in]
        n5073 = call-dynamic "Write target.vi"("error in (no error)"=w12183, "target"=w12173, "GSdevice in"=w12184) -> ("error out"=w12180:errorcluster, "GSdevice out"=w12182:refnum<class "GSdevice.lvclass">)  [unwired: 7 in]
